vi "Update Run Listen Button.vi"(8 "error in (no error)":errorcluster, 9 "Use First Entry":bool, 10 "Plugin Filter":string, 11 "CIFManager_UI in":refnum<class "CIF_UI.lvclass">) -> (0 "error out":errorcluster)   [LabVIEW 2021, in "CIF_UI.lvclass"]
uses:
  CIF_UI.lvclass
  CIF_UI.lvclass/CIF_UI.ctl
  CIFCore/Common/Typedef/Plugin State.ctl
  CIFCore/Common/CIFCoreCommon.lvlib
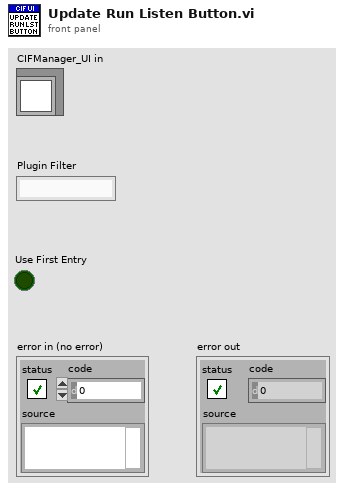
[diagram p1: front panel]
types:
  T1 = typedef "CIFCoreCommon.lvlib/Plugin State.ctl" = enum32{"Null", "Creating", "Listening", "Running", "CleaningUp", "Destroying"}
  T2 = typedef "CIF_UI.lvclass/Plugin Connection Map.ctl" = map{string, T3}
  T3 = typedef "CIF_UI.lvclass/Plugin Connections.ctl" = cluster{"gRPC ID":T4, "Plugin Info":T5}
  T4 = typedef "grpc-lvsupport-release.lvlib/grpcId.ctl" = u64
  T5 = typedef "CIF_UI.lvclass/PluginInfo.ctl" = cluster{"Name":string, "Type":string, "grpc_port":i32, "Version":T6, "Node Status":T7}
  T6 = typedef "CIF_UI.lvclass/Version.ctl" = cluster{"Major":i32, "Minor":i32, "Fix":i32}
  T7 = typedef "CIFCoreCommon.lvlib/gRPC Reported Plugin Status.ctl" = cluster{"State":T1, "Timing Statistics (us)":T8, "FIFO Statistics (us)":T10, "error":T11, "Monitor Doubles":T12, "Monitor U64":T13, "Monitor I64":T14}
  T8 = typedef "CIFCoreCommon.lvlib/Timing Statistics.ctl" = cluster{"Period":T9, "Wake Error":T9, "Execute":T9, "Housekeep":T9, "Idle":T9, "Cleanup":T9, "Custom 1 (custom units)":T9, "Custom 2 (custom units)":T9}
  T9 = typedef "CIFCoreCommon.lvlib/Timing Stats Base.ctl" = cluster{"Max":i64, "Avg":dbl, "Min":i64}
  T10 = typedef "CIFCoreCommon.lvlib/FIFO Statistics.ctl" = cluster{"From T0":T9, "From Previous Plugin":T9, "Output Error":T9}
  T11 = typedef "CIFCoreCommon.lvlib/Simple Error.ctl" = cluster{"status":bool, "code":i32}
  T12 = typedef "CIFCoreCommon.lvlib/Monitor Doubles.ctl" = cluster{"1":dbl, "2":dbl, "3":dbl, "4":dbl}
  T13 = typedef "CIFCoreCommon.lvlib/Monitor U64.ctl" = cluster{"1":u64, "2":u64, "3":u64, "4":u64}
  T14 = typedef "CIFCoreCommon.lvlib/Monitor I64.ctl" = cluster{"1":i64, "2":i64, "3":i64, "4":i64}
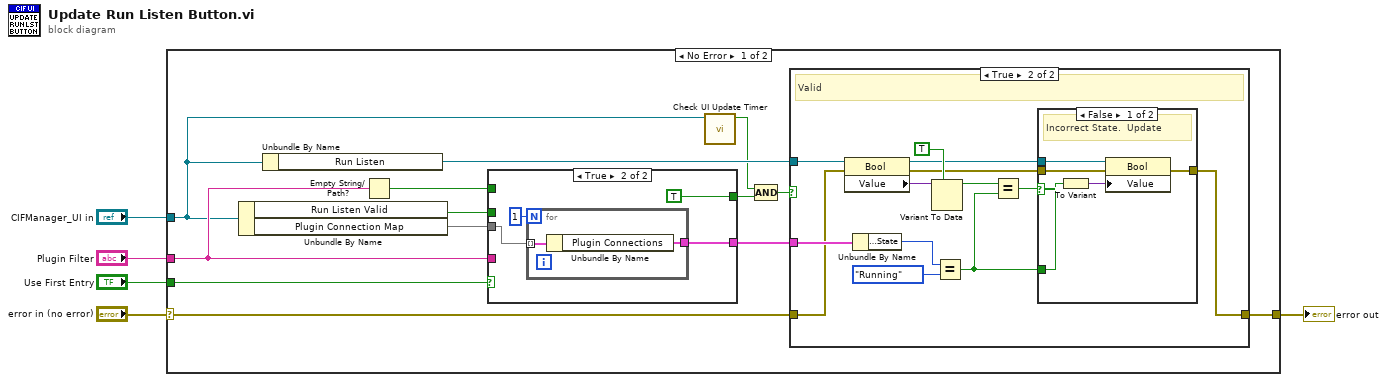
[diagram p0: block diagram]
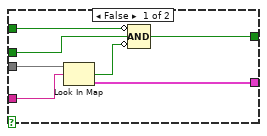
[diagram p2: hidden frame]
diagram:
  n1 = case shown="No Error" "error in (no error)" {
    selector: "error in (no error)" -> [w18 w52]
    tunnel: [w12 w52] -> w4
    tunnel: "CIFManager_UI in" -> [w9 _]
    tunnel: "Plugin Filter" -> [w14 _]
    tunnel: "Use First Entry" -> [w11 _]
    frame No Error {
      n2 = Unbundle By Name(w9) -> ("Run Listen Valid"=w17:bool, "Plugin Connection Map"=w15:T2)
      n3 = Unbundle By Name(w9) -> ("Run Listen"=w10:refnum<vi>)
      n4 = Empty String/Path?(string/path=w14) -> (empty?=w16:bool)
      n5 = case shown="True" w11 {
        tunnel: w17 -> [w25 _]
        tunnel: w16 -> [w24 _]
        tunnel: [w23 TRUE] -> w8
        tunnel: w15 -> [w22 w29]
        tunnel: w14 -> [w21 _]
        tunnel: [w19 w27] -> w13
        frame False {
          n6 = Look In Map(map=w22, key=w21) -> (key not found?=w20:bool, value=w19:T3)  [unwired: 1 in]
          n7 = Compound Arithmetic op=AND(invert w24, w25, invert w20) -> (w23:bool)
        }
        frame True {
          n8 = for {
            N: 1 -> [_]
            tunnel: w29 -> [w31] mode=indexing
            tunnel: [w30] -> w27
            n9 = Unbundle By Name(w31) -> ("Plugin Connections"=w30:T3)
          }
        }
      }
      n10 = call "Check UI Update Timer.vi"("CIF_UI in"=w9) -> ("Timeout"=w6:bool)  [unwired: 10 in]
      n11 = Compound Arithmetic op=AND(w6, w8) -> (w7:bool)
      n12 = case shown="True" w7 {
        tunnel: w10 -> [_ w42]
        tunnel: w13 -> [_ w45]
        tunnel: w18 -> [w32 w34]
        tunnel: [w32 w33] -> w12
        frame False {
        }
        frame True {
          # "Valid"
          n13 = property class="Bool"(reference=w42, error in=w34) -> (reference out=w37:refnum<vi>, error out=w35:errorcluster, "Value"=w41:variant)
          n14 = Unbundle By Name(w45) -> ("Plugin Info.Node Status.State"=w44:T1)
          n15 = Variant To Data(type=TRUE, Variant=w41) -> (data=w39:bool)  [unwired: 1 in, 1 out]
          n16 = Equal?(x=w44, y=Plugin_State."Running") -> (x = y?=w36:bool)
          n17 = Equal?(x=w39, y=w36) -> (x = y?=w38:bool)
          n18 = case shown="False" w38 {
            tunnel: w37 -> [w50 _]
            tunnel: w36 -> [w49 _]
            tunnel: w35 -> [w48 w51]
            tunnel: [w47 w51] -> w33
            frame False {
              # "Incorrect State.  Update"
              n19 = To Variant(anything=w49) -> (Variant=w46:variant)
              n20 = property class="Bool"(reference=w50, error in=w48, "Value"=w46) -> (error out=w47:errorcluster)  [unwired: 1 out]
            }
            frame True {
              # "Correct State"
            }
          }
        }
      }
    }
    frame Error {
    }
  }
  "error out" <- w4
